vi "3-3.vi"() -> ()   [LabVIEW 2022 SP3]
panel:
  in  "Y":dbl[](array[numeric])
  in  "X":dbl[](array[numeric])
  out "XY Graph":cluster{"Y":dbl[], "Y":dbl[]}[](graph) caption="XY图"
  out "XY图":cluster{"X":dbl[], "Y":dbl[]}(graph)
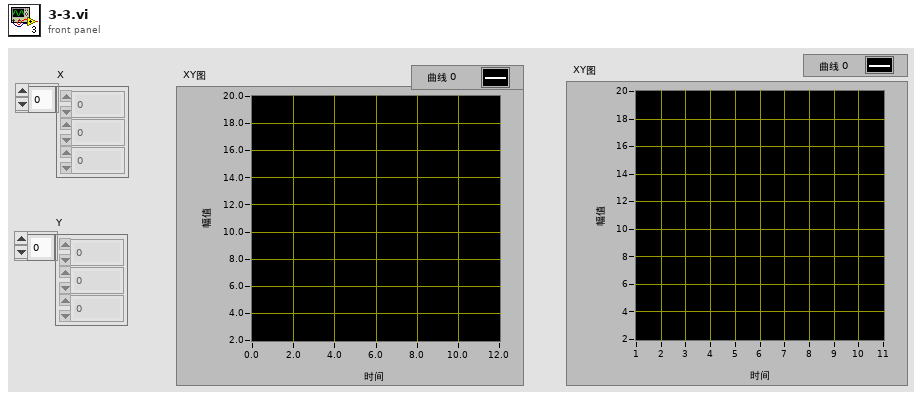
[diagram p1: front panel]
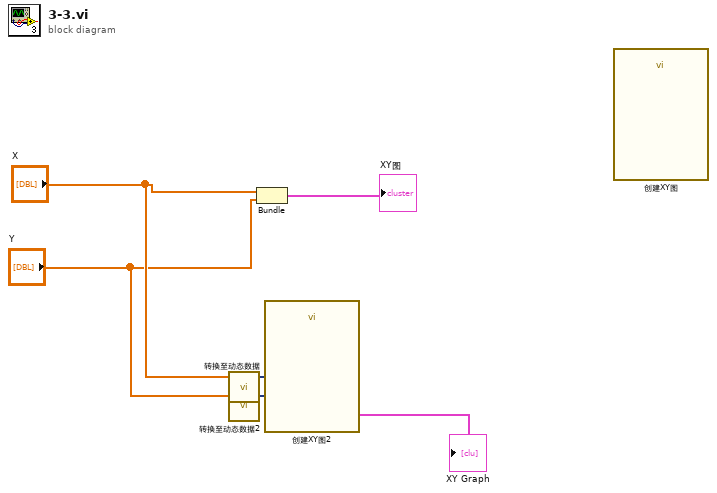
[diagram p0: block diagram]
diagram:
  n1 = call "转换至动态数据"("Array"="X") -> ("Dynamic Data Type"=w3:dynamicdata)  [unwired: 3 in]
  n2 = call "转换至动态数据2"("Array"="Y") -> ("Dynamic Data Type"=w1:dynamicdata)  [unwired: 3 in]
  n3 = Bundle("X"="X", "Y"="Y") -> (→"XY图":cluster{"X":dbl[], "Y":dbl[]})  [unwired: 1 in]
  n4 = call "创建XY图2"("Y Input"=w1, "X Input"=w3) -> ("XY Graph"=→"XY Graph":cluster{"X":dbl[], "Y":dbl[]}[])  [unwired: 8 in, 1 out]
  n5 = call "创建XY图"() -> ()  [unwired: 10 in, 2 out]
